vi "Teleop.vi"(10 "Match Info":T1={"Autonomous Elapsed Seconds"=0.0, "TeleOp Elapsed Seconds"=0.0, "Disabled Elapsed Seconds"=0.0, "Visited Autonomous"=FALSE, "Visited TeleOp"=FALSE, "Visited Disabled"=FALSE, "Autonomous Settings"={"Autonomous Style"=enum."Independent", "VI Refnum"=refnum}}, 11 "Call Context":T2) -> ()   [LabVIEW 2013]
doc: "This VI is called for each TeleOp packet received from the DS where the robot is not disabled. It is often used to read from the joysticks and update I/O or to update setpoints for timed control loops. It should complete and return within 20 milliseconds or it may miss DS packets."
uses:
  <vilib>/Rock Robotics/WPI/DriverStation/WPI_DriverStationDerivedRobotMode.ctl
  <vilib>/Rock Robotics/WPI/DriverStation/WPI_DriverStationMatch Info.ctl
  <vilib>/Rock Robotics/WPI/Relay/WPI_RelayValue.ctl
  <vilib>/Rock Robotics/WPI/Solenoid/WPI_SolenoidValue.ctl
  Robot Global Data.vi
  <vilib>/Rock Robotics/WPI/Solenoid/WPI_SolenoidSetEnum.vi
  <vilib>/Rock Robotics/WPI/Joystick/WPI_JoystickGetSetRefNum.vi
  <vilib>/Rock Robotics/WPI/RobotDrive/WPI_RobotDriveGetSetRefNum.vi
panel:
  out "Numeric 1":dbl(slide) scale=0.0..100.0
  out "Boolean 2":bool
  out "Boolean 1":bool
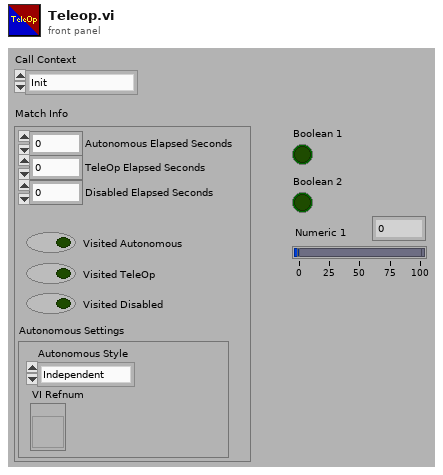
[diagram p1: front panel]
types:
  T1 = typedef "WPI_DriverStationMatch Info.ctl" = cluster{"Autonomous Elapsed Seconds":dbl, "TeleOp Elapsed Seconds":dbl, "Disabled Elapsed Seconds":dbl, "Visited Autonomous":bool, "Visited TeleOp":bool, "Visited Disabled":bool, "Autonomous Settings":cluster{"Autonomous Style":enum16{"Iterative", "Independent"}, "VI Refnum":refnum<vi>}}
  T2 = typedef "WPI_DriverStationDerivedRobotMode.ctl" = enum16{"Init", "Execute", "Stop"}
  T3 = typedef "WPI_RelayValue.ctl" = enum16{"Off", "On", "Forward", "Reverse"}
  T4 = typedef "WPI_AnalogChannelDevRef.ctl" = cluster{"DevStatus":errorcluster, "Analog Module":T5, "Analog Channel":T6}
  T5 = typedef "FPGA_TypedefAnalogModule.ctl" = enum16{"Analog Module 1", "Analog Module 2"}
  T6 = typedef "FPGA_AIChannel.ctl" = enum8{"AI 1", "AI 2", "AI 3", "AI 4", "AI 5", "AI 6", "AI 7", "AI 8", "Invalid"}
  T7 = typedef "WPI_JoystickDevRef.ctl" = cluster{"Device":T8}
  T8 = typedef "WPI_JoystickDeviceEnum.ctl" = enum16{"USB 1", "USB 2", "USB 3", "USB 4", "Kinect 1", "Kinect 2"}
  T9 = typedef "WPI_JoystickButtonState.ctl" = cluster{"Button 1":bool, "Button 2":bool, "Button 3":bool, "Button 4":bool, "Button 5":bool, "Button 6":bool, "Button 7":bool, "Button 8":bool, "Button 9":bool, "Button 10":bool, "Button 11":bool, "Button 12":bool}
  T10 = cluster{"axis 1 (x)":dbl, "axis 2 (y)":dbl, "axis 3 (throttle)":dbl, "axis 4":dbl, "axis 5":dbl, "axis 6":dbl}
  T11 = typedef "WPI_SolenoidDevRef.ctl" = cluster{"DevStatus":errorcluster, "Solenoid Module":T12, "Forward Solenoid Channel":T13, "Reverse Solenoid Channel":T13}
  T12 = typedef "FPGA_TypedefSolenoidModule.ctl" = enum16{"Solenoid Module 1", "Solenoid Module 2"}
  T13 = typedef "WPI_SolenoidChannel.ctl" = enum8{"Solenoid 1", "Solenoid 2", "Solenoid 3", "Solenoid 4", "Solenoid 5", "Solenoid 6", "Solenoid 7", "Solenoid 8", "Invalid"}
  T14 = typedef "WPI_MotorControlDeviceRef.ctl" = cluster{"DeviceStatus":errorcluster, "Type":enum16{"PWM", "CAN"}, "PWM":cluster{"Digital Module":T15, "PWM Channel":T16, "DeadBand":T17}, "CAN":cluster{"Device Number":u8, "Control Mode":T18, "Semaphore":T19, "Max Vout":dbl}, "Invert":bool, "TransformRef":T20, "InvTransformRef":T20}
  T15 = typedef "FPGA_TypedefDigitalModule.ctl" = enum16{"Digital Module 1", "Digital Module 2"}
  T16 = typedef "FPGA_DIOPWMChannel.ctl" = enum8{"PWM 1", "PWM 2", "PWM 3", "PWM 4", "PWM 5", "PWM 6", "PWM 7", "PWM 8", "PWM 9", "PWM 10", "Invalid"}
  T17 = typedef "WPI_PWMDeadband.ctl" = cluster{"Name":string, "maxPositivePwm":i32, "minPositivePwm":i32, "centerPwm":i32, "maxNegativePwm":i32, "minNegativePwm":i32, "angularRange":u16}
  T18 = typedef "WPI_CANJaguar_ControlMode.ctl" = enum8{"Percent VBus", "Current", "Speed", "Position", "Voltage"}
  T19 = typedef "Semaphore RefNum" = refnum<k1>
  T20 = typedef "WPI_PWMTransform_ConPane.ctl" = refnum<vi>
  T21 = typedef "WPI_SolenoidValue.ctl" = enum16{"Off", "On", "Forward", "Reverse"}
  T22 = typedef "WPI_RelayDevRef.ctl" = cluster{"DevStatus":errorcluster, "Relay Channel":T23, "Digital Module":T15, "Relay Direction":T24}
  T23 = typedef "FPGA_DIORelayChannel.ctl" = enum8{"Relay 1", "Relay 2", "Relay 3", "Relay 4", "Relay 5", "Relay 6", "Relay 7", "Relay 8", "Invalid"}
  T24 = typedef "WPI_RelayDirection.ctl" = enum16{"Both directions", "Forward only", "Reverse only"}
  T25 = typedef "WPI_RobotDriveDevRef.ctl" = cluster{"DevStatus":errorcluster, "Motors[]":T14[], "Square Inputs":bool, "Max Output":dbl, "Isochronous":bool}
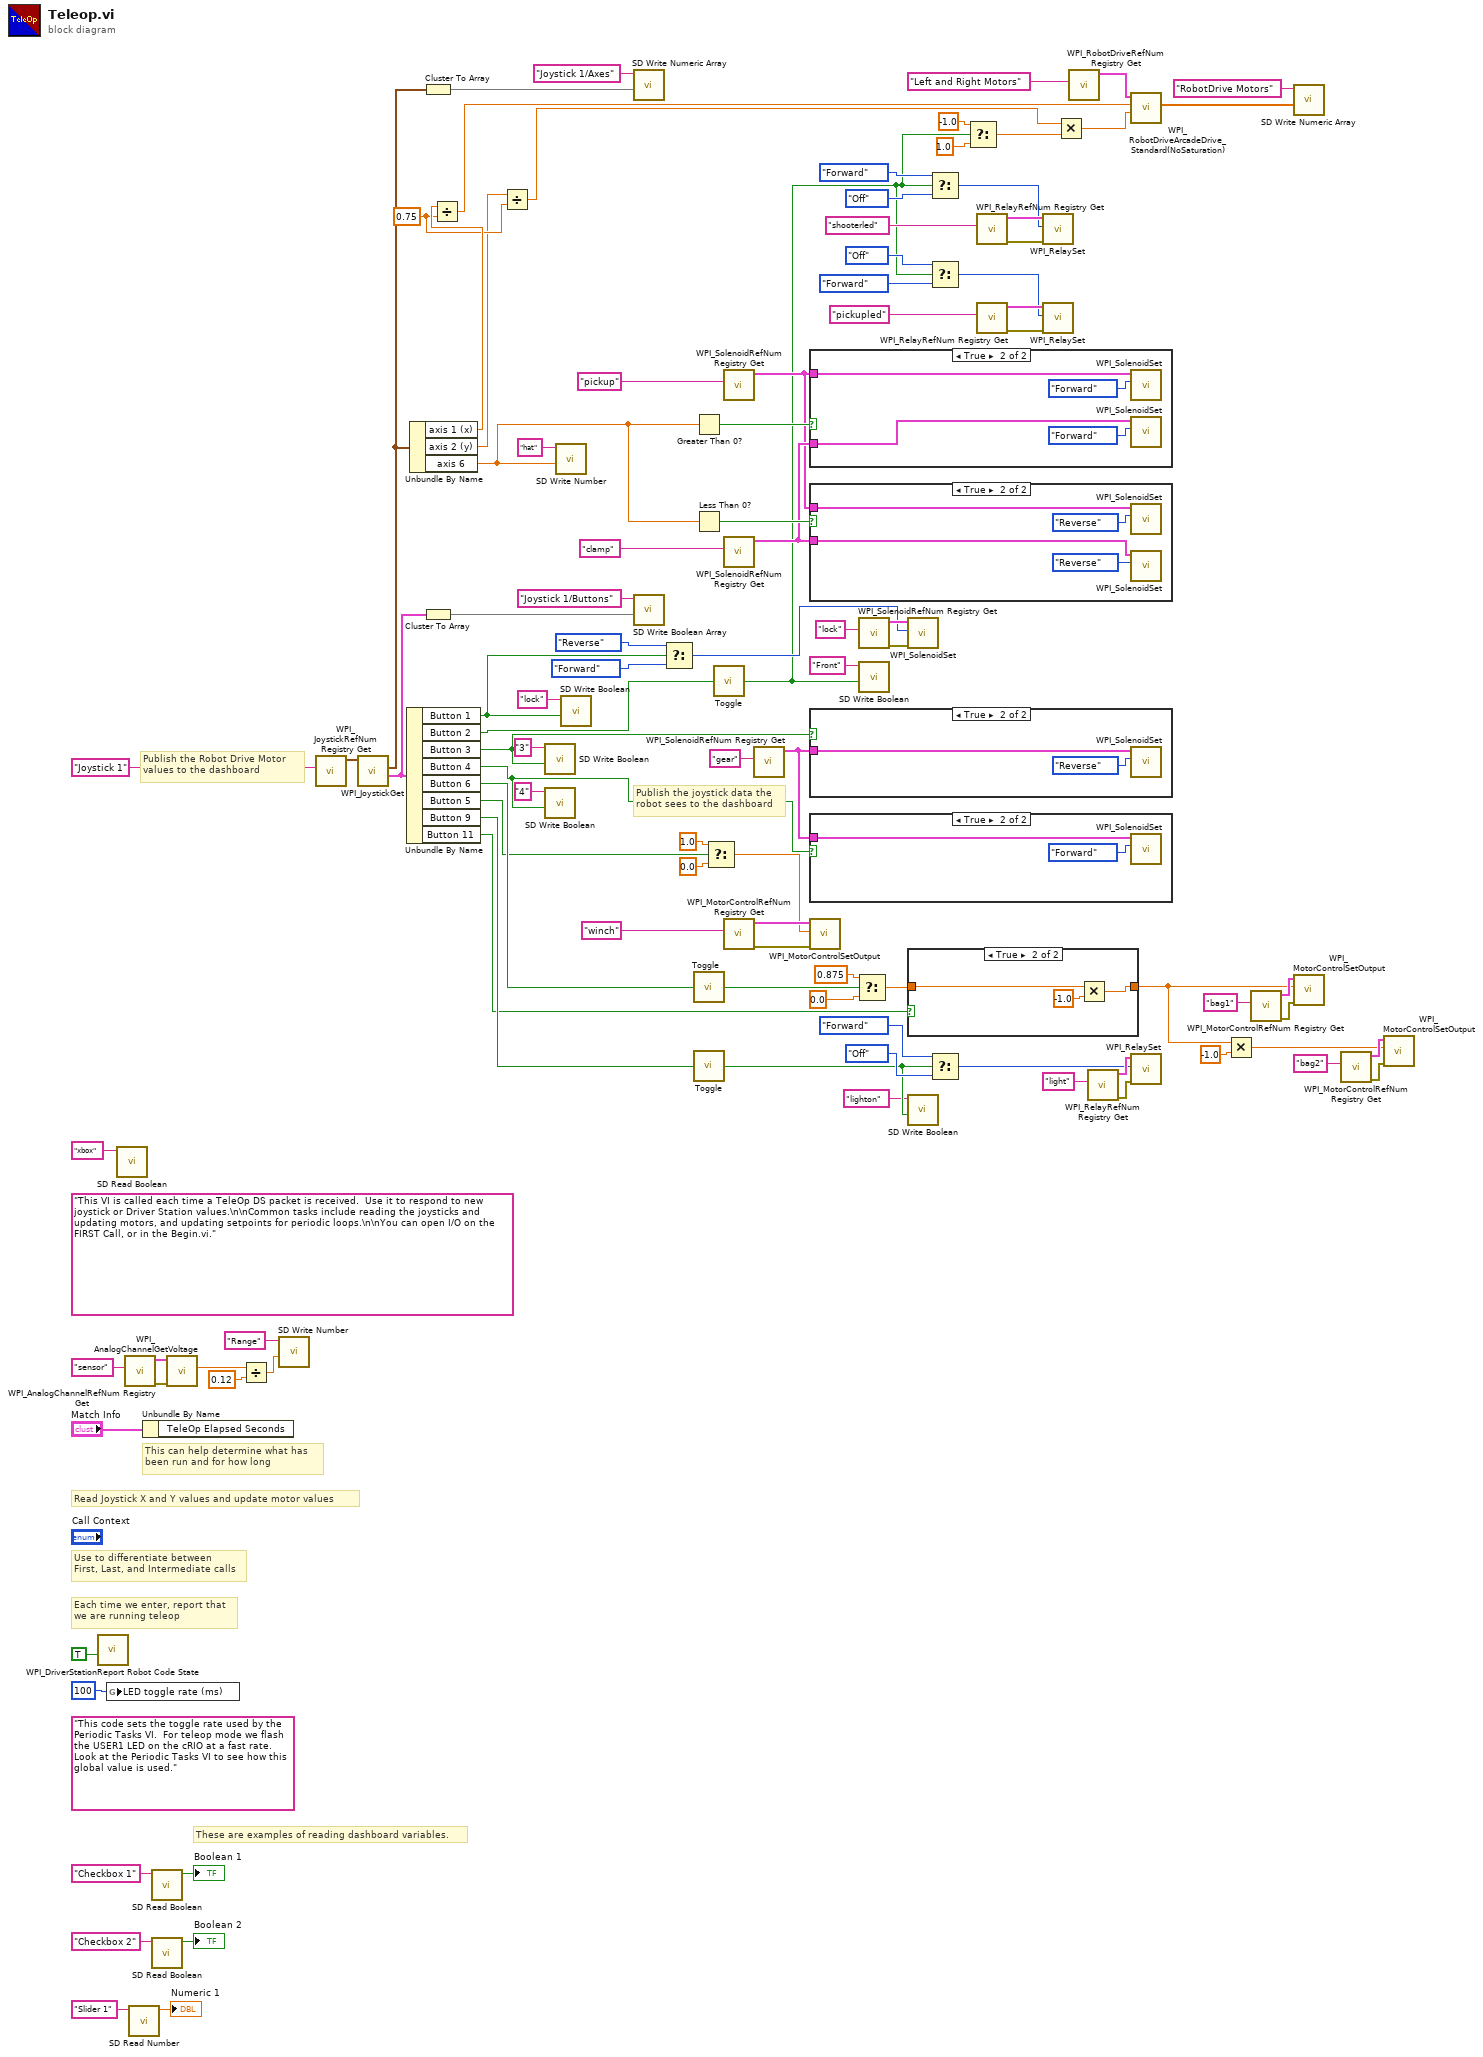
[diagram p0: block diagram]
diagram:
  w2 = 0.75 ("y")
  (unwired) "This code sets the toggle rate used by the Periodic Tasks VI.  For teleop mode we flash the USER1 LED on the cRIO at a fast rate.  Look at the Periodic Tasks VI to see how this global value is used."
  (unwired) "This VI is called each time a TeleOp DS packet is received.  Use it to respond to new joystick or Driver Station values.\n\nCommon tasks include reading the joysticks and updating motors, and updating setpoints for periodic loops.\n\nYou can open I/O on the FIRST Call, or in the Begin.vi."
  # "Publish the joystick data the\nrobot sees to the dashboard"
  # "Publish the Robot Drive Motor\nvalues to the dashboard"
  # "These are examples of reading dashboard variables."
  # "Each time we enter, report that\nwe are running teleop"
  # "Use to differentiate between\nFirst, Last, and Intermediate calls"
  # "This can help determine what has\nbeen run and for how long"
  # "Read Joystick X and Y values and update motor values"
  n1 = call <vilib>:"WPI_DriverStationReport Robot Code State.vi"("TeleOp"=TRUE ("Autonomous")) -> ()  [unwired: 10 in, 1 out]
  n2 = global write "Robot Global Data.vi" "LED toggle rate (ms)"(u32 100 ("LED ms toggle rate")) -> ()
  n3 = call <vilib>:"SD Read Boolean.vi"("Name"="xbox") -> ()  [unwired: 8 in, 3 out]
  n4 = call <vilib>:"WPI_AnalogChannelRefNum Registry Get.vi"("refnum name"="sensor") -> ("error out"=w90:errorcluster, "AIDeviceRef"=w91:T4)  [unwired: 9 in]
  n5 = call <vilib>:"SD Read Number.vi"("Name"="Slider 1" ("refnum name")) -> ("Numeric"=→"Numeric 1":dbl)  [unwired: 8 in, 2 out]
  n6 = Unbundle By Name("Match Info") -> ()  [unwired: 1 out]
  n7 = call <vilib>:"SD Read Boolean.vi"("Name"="Checkbox 1" ("refnum name")) -> ("Boolean"=→"Boolean 1":bool)  [unwired: 8 in, 2 out]
  n8 = call <vilib>:"SD Read Boolean.vi"("Name"="Checkbox 2" ("refnum name")) -> ("Boolean"=→"Boolean 2":bool)  [unwired: 8 in, 2 out]
  n9 = call <vilib>:"WPI_AnalogChannelGetVoltage.vi"("error in (no error)"=w90, "AIDeviceRef"=w91) -> ("Voltage"=w88:dbl)  [unwired: 7 in, 2 out]
  n10 = Divide(x=w88, y=0.12) -> (x/y=w86:dbl)
  n11 = call <vilib>:"SD Write Number.vi"("Numeric"=w86, "Name"="Range") -> ()  [unwired: 8 in, 2 out]
  n12 = call <vilib>:"WPI_JoystickRefNum Registry Get.vi"("refnum name"="Joystick 1") -> ("JoystickDevRef"=w104:T7)  [unwired: 1 in, 9 out]
  n13 = call <vilib>:"WPI_JoystickGet.vi"("JoystickDevRef"=w104) -> ("Buttons"=w83:T9, "Axes"=w84:T10)  [unwired: 1 in, 4 out]
  n14 = Unbundle By Name(w83) -> ("Button 1"=w34:bool, "Button 2"=w77:bool, "Button 3"=w28:bool, "Button 4"=w27:bool, "Button 6"=w35:bool, "Button 5"=w9:bool, "Button 9"=w16:bool, "Button 11"=w10:bool)
  n15 = Unbundle By Name(w84) -> ("axis 1 (x)"=w4:dbl, "axis 2 (y)"=w1:dbl, "axis 6"=w32:dbl)
  n16 = Cluster To Array(cluster=w84) -> (array=w99:dbl[])
  n17 = Cluster To Array(cluster=w83) -> (array=w101:bool[])
  n18 = Divide(x=w4, y=w2) -> (x/y=w5:dbl)
  n19 = Divide(x=w1, y=w2) -> (x/y=w3:dbl)
  n20 = call <vilib>:"SD Write Boolean.vi"("Boolean"=w28, "Name"="3") -> ()  [unwired: 8 in, 2 out]
  n21 = call <vilib>:"SD Write Boolean.vi"("Boolean"=w27, "Name"="4") -> ()  [unwired: 8 in, 2 out]
  n22 = call <vilib>:"SD Write Number.vi"("Numeric"=w32, "Name"="hat") -> ()  [unwired: 8 in, 2 out]
  n23 = call <vilib>:"SD Write Boolean.vi"("Boolean"=w34, "Name"="lock") -> ()  [unwired: 8 in, 2 out]
  n24 = call <vilib>:"SD Write Numeric Array.vi"("Numeric Array"=w99, "Name"="Joystick 1/Axes") -> ()  [unwired: 8 in, 2 out]
  n25 = call <vilib>:"SD Write Boolean Array.vi"("Boolean Array"=w101, "Name"="Joystick 1/Buttons") -> ()  [unwired: 8 in, 2 out]
  n26 = Select(t=WPI_RelayValue."Reverse" ("RelayValue"), s=w34, f=WPI_RelayValue."Forward") -> (s? t:f=w50:T3)
  n27 = Greater Than 0?(x=w32) -> (x > 0?=w61:bool)
  n28 = Less Than 0?(x=w32) -> (x < 0?=w62:bool)
  n29 = call "Toggle.vi"("Input"=w35) -> ("Output"=w41:bool)
  n30 = call "Toggle.vi"("Input"=w16) -> ("Output"=w15:bool)
  n31 = Select(t=1.0, s=w9, f=0.0) -> (s? t:f=w8:dbl)
  n32 = call "Toggle.vi"("Input"=w77) -> ("Output"=w37:bool)
  n33 = call <vilib>:"WPI_SolenoidRefNum Registry Get.vi"("refnum name"="pickup") -> ("SolenoidDevRef"=w57:T11)  [unwired: 9 in, 1 out]
  n34 = call <vilib>:"WPI_SolenoidRefNum Registry Get.vi"("refnum name"="clamp") -> ("SolenoidDevRef"=w58:T11)  [unwired: 9 in, 1 out]
  n35 = call <vilib>:"WPI_MotorControlRefNum Registry Get.vi"("refnum name"="winch") -> ("error out"=w12:errorcluster, "MotorControlDevRef"=w13:T14)  [unwired: 9 in]
  n36 = call <vilib>:"WPI_SolenoidRefNum Registry Get.vi"("refnum name"="gear") -> ("SolenoidDevRef"=w55:T11)  [unwired: 9 in, 1 out]
  n37 = case shown="True" w61 {
    tunnel: w58 -> [_ w110]
    tunnel: w57 -> [_ w109]
    frame False {
    }
    frame True {
      n38 = call-poly <vilib>:"WPI_SolenoidSet.vi"("Value"=WPI_SolenoidValue."Forward", "SolenoidDevRef"=w109) -> ()  [unwired: 8 in, 2 out]
      n39 = call-poly <vilib>:"WPI_SolenoidSet.vi"("Value"=WPI_SolenoidValue."Forward", "SolenoidDevRef"=w110) -> ()  [unwired: 8 in, 2 out]
    }
  }
  n40 = case shown="True" w62 {
    tunnel: w58 -> [_ w114]
    tunnel: w57 -> [_ w113]
    frame False {
    }
    frame True {
      n41 = call-poly <vilib>:"WPI_SolenoidSet.vi"("Value"=WPI_SolenoidValue."Reverse", "SolenoidDevRef"=w113) -> ()  [unwired: 8 in, 2 out]
      n42 = call-poly <vilib>:"WPI_SolenoidSet.vi"("Value"=WPI_SolenoidValue."Reverse", "SolenoidDevRef"=w114) -> ()  [unwired: 8 in, 2 out]
    }
  }
  n43 = case shown="True" w28 {
    tunnel: w55 -> [_ w115]
    frame False {
    }
    frame True {
      n44 = call-poly <vilib>:"WPI_SolenoidSet.vi"("Value"=WPI_SolenoidValue."Reverse", "SolenoidDevRef"=w115) -> ()  [unwired: 8 in, 2 out]
    }
  }
  n45 = case shown="True" w27 {
    tunnel: w55 -> [_ w117]
    frame False {
    }
    frame True {
      n46 = call-poly <vilib>:"WPI_SolenoidSet.vi"("Value"=WPI_SolenoidValue."Forward", "SolenoidDevRef"=w117) -> ()  [unwired: 8 in, 2 out]
    }
  }
  n47 = call <vilib>:"WPI_MotorControlSetOutput.vi"("error in (no error)"=w12, "Output"=w8, "MotorControlDevRef"=w13) -> ()  [unwired: 6 in, 3 out]
  n48 = Select(t=0.875, s=w41, f=0.0) -> (s? t:f=w29:dbl)
  n49 = call <vilib>:"WPI_SolenoidRefNum Registry Get.vi"("refnum name"="lock") -> ("error out"=w53:errorcluster, "SolenoidDevRef"=w54:T11)  [unwired: 9 in]
  n50 = call <vilib>:"SD Write Boolean.vi"("Boolean"=w37, "Name"="Front") -> ()  [unwired: 8 in, 2 out]
  n51 = call-poly <vilib>:"WPI_SolenoidSet.vi"("error in (no error)"=w53, "Value"=w50, "SolenoidDevRef"=w54) -> ()  [unwired: 7 in, 2 out]
  n52 = case shown="True" w10 {
    tunnel: [w119 w120] -> w30
    tunnel: w29 -> [w119 w121]
    frame False {
    }
    frame True {
      n53 = Multiply(x=w121, y=-1.0) -> (x*y=w120:dbl)
    }
  }
  n54 = call <vilib>:"SD Write Boolean.vi"("Boolean"=w15, "Name"="lighton") -> ()  [unwired: 8 in, 2 out]
  n55 = Select(t=WPI_RelayValue."Forward" ("RelayValue"), s=w37, f=WPI_RelayValue."Off") -> (s? t:f=w24:T3)
  n56 = Select(t=WPI_RelayValue."Off" ("RelayValue"), s=w37, f=WPI_RelayValue."Forward") -> (s? t:f=w23:T3)
  n57 = Select(t=WPI_RelayValue."Forward" ("RelayValue"), s=w15, f=WPI_RelayValue."Off") -> (s? t:f=w17:T3)
  n58 = Select(t=-1.0, s=w37, f=1.0) -> (s? t:f=w66:dbl)
  n59 = call <vilib>:"WPI_RelayRefNum Registry Get.vi"("refnum name"="shooterled") -> ("error out"=w71:errorcluster, "RelayDevRef"=w70:T22)  [unwired: 9 in]
  n60 = call <vilib>:"WPI_RelayRefNum Registry Get.vi"("refnum name"="pickupled") -> ("error out"=w76:errorcluster, "RelayDevRef"=w75:T22)  [unwired: 9 in]
  n61 = call <vilib>:"WPI_RelaySet.vi"("error in (no error)"=w71, "RelayValue"=w24, "RelayDevRef"=w70) -> ()  [unwired: 7 in, 2 out]
  n62 = call <vilib>:"WPI_RelaySet.vi"("error in (no error)"=w76, "RelayValue"=w23, "RelayDevRef"=w75) -> ()  [unwired: 7 in, 2 out]
  n63 = Multiply(x=w3, y=w66) -> (x*y=w65:dbl)
  n64 = call <vilib>:"WPI_RobotDriveRefNum Registry Get.vi"("refnum name"="Left and Right Motors") -> ("RobotDriveDevRef"=w80:T25)  [unwired: 1 in, 9 out]
  n65 = call <vilib>:"WPI_RelayRefNum Registry Get.vi"("refnum name"="light") -> ("error out"=w21:errorcluster, "RelayDevRef"=w22:T22)  [unwired: 9 in]
  n66 = call <vilib>:"WPI_RobotDriveArcadeDrive_Standard(NoSaturation).vi"("Y axis value"=w65, "X axis value"=w5, "RobotDriveDevRef"=w80) -> ("Motor Values"=w78:dbl[])  [unwired: 1 in, 7 out]
  n67 = call <vilib>:"WPI_RelaySet.vi"("error in (no error)"=w21, "RelayValue"=w17, "RelayDevRef"=w22) -> ()  [unwired: 7 in, 2 out]
  n68 = Multiply(x=w30, y=-1.0) -> (x*y=w40:dbl)
  n69 = call <vilib>:"WPI_MotorControlRefNum Registry Get.vi"("refnum name"="bag1") -> ("error out"=w44:errorcluster, "MotorControlDevRef"=w45:T14)  [unwired: 9 in]
  n70 = call <vilib>:"SD Write Numeric Array.vi"("Numeric Array"=w78, "Name"="RobotDrive Motors") -> ()  [unwired: 8 in, 2 out]
  n71 = call <vilib>:"WPI_MotorControlSetOutput.vi"("error in (no error)"=w44, "Output"=w30, "MotorControlDevRef"=w45) -> ()  [unwired: 6 in, 3 out]
  n72 = call <vilib>:"WPI_MotorControlRefNum Registry Get.vi"("refnum name"="bag2") -> ("error out"=w47:errorcluster, "MotorControlDevRef"=w48:T14)  [unwired: 9 in]
  n73 = call <vilib>:"WPI_MotorControlSetOutput.vi"("error in (no error)"=w47, "Output"=w40, "MotorControlDevRef"=w48) -> ()  [unwired: 6 in, 3 out]
